vi "Vector3DtoVector2D_XZ.vi"(10 "Vector3D":T2) -> (2 "Vector2D":T1)   [LabVIEW 2018]
uses:
  Vector3D.ctl
  Vector2D.ctl
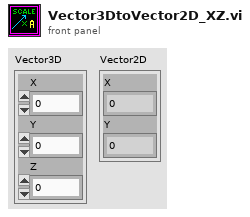
[diagram p1: front panel]
types:
  T1 = typedef "Vector2D.ctl" = cluster{"X":dbl, "Y":dbl}
  T2 = typedef "Vector3D.ctl" = cluster{"X":dbl, "Y":dbl, "Z":dbl}
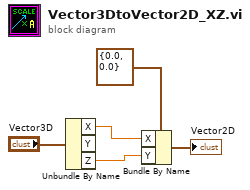
[diagram p0: block diagram]
diagram:
  n1 = Unbundle By Name("Vector3D") -> ("X"=w1:dbl, "Z"=w2:dbl)  [unwired: 1 out]
  n2 = Bundle By Name(cluster=T1 {"X"=0.0, "Y"=0.0} ("Vector2D 2"), "X"=w1, "Y"=w2) -> (→"Vector2D":T1)
